vi "DS345_BurstMode.ProcCases.vi"(0 "i ref in":refnum<vi>, 1 "selector":string, 2 "Data":T1, 3 "call cluster":T2={"Object"="", "Selector"="", "CallType"=enum."synchronous", "Async Object"="", "Async Selector"="", "Data Descriptor"="", "Data"=[], "Error #"=0, "Expire"=0}, 5 "error in (no error)":errorcluster) -> (14 "i ref out":refnum<vi>, 17 "answer cluster":T2={"Object"="", "Selector"="", "CallType"=enum."synchronous", "Async Object"="", "Async Selector"="", "Data Descriptor"="", "Data"=[], "Error #"=0, "Expire"=0}, 19 "error out":errorcluster)   [LabVIEW 2014, in "DS345_BurstMode.lvlib"]
doc: "This method is called by a process from within the default case in the event loop. The methods of a class that are linked to events will be called from THIS method. Add your code here."
uses:
  DS345_BurstMode.lvlib
  CS_Core/CSSystem/CoreDefs/CoreDefs.call_type.ctl
  CS_Core/BaseProcess/BaseProcess.descriptor string definition.ctl
  CS_Core/CSSystem/CoreDefs/CoreDefs.rawDataType.ctl
  CS_Core/CSSystem/CoreLib/CoreLib.string 2 byte array.vi
  CS_Core/CSSystem/CoreLib/CoreLib.byte array 2 double.vi
  CS_Core/CSSystem/CoreLib/CoreLib.double 2 byte array.vi
  CS_Core/CSSystem/CoreLib/CoreLib.lvlib
  CS_Core/BaseProcess/BaseProcess.lvlib
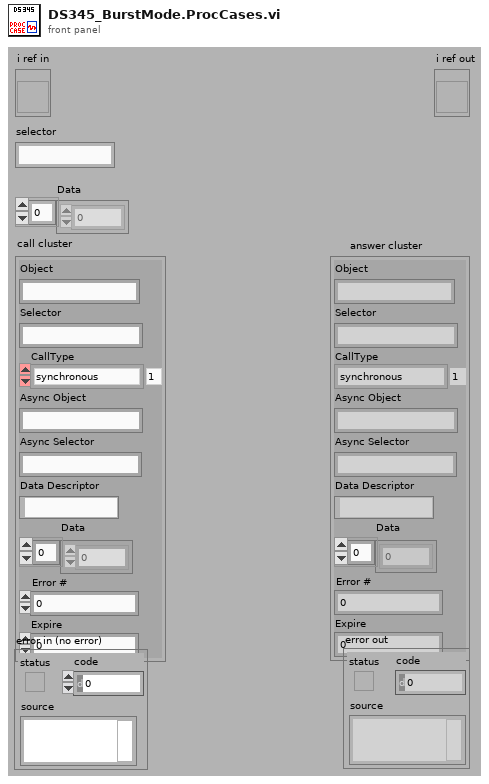
[diagram p1: front panel]
types:
  T1 = typedef "CoreDefs.rawDataType.ctl" = i8[]
  T2 = typedef "CoreDefs.call_type.ctl" = cluster{"Object":string, "Selector":string, "CallType":enum16{"simple", "synchronous", "asynchronous"}, "Async Object":string, "Async Selector":string, "Data Descriptor":T3, "Data":T1, "Error #":i32, "Expire":u32}
  T3 = typedef "BaseProcess.lvlib/BaseProcess.descriptor string definition.ctl" = string
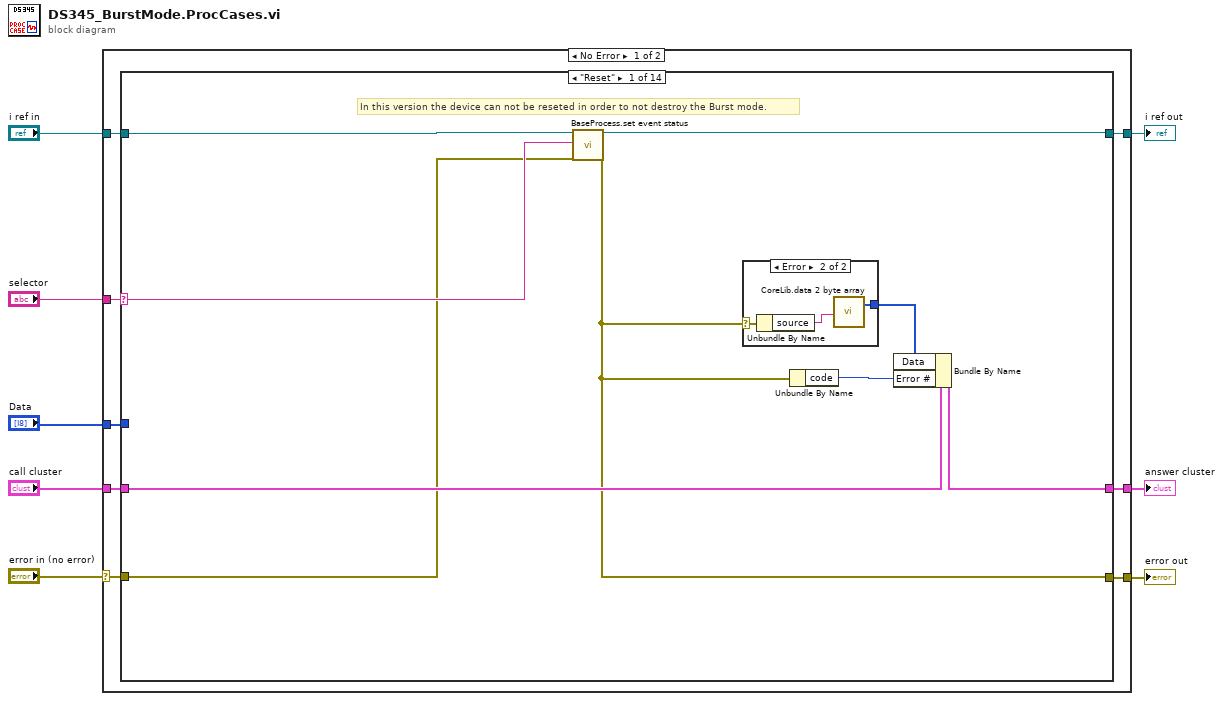
[diagram p0: block diagram]
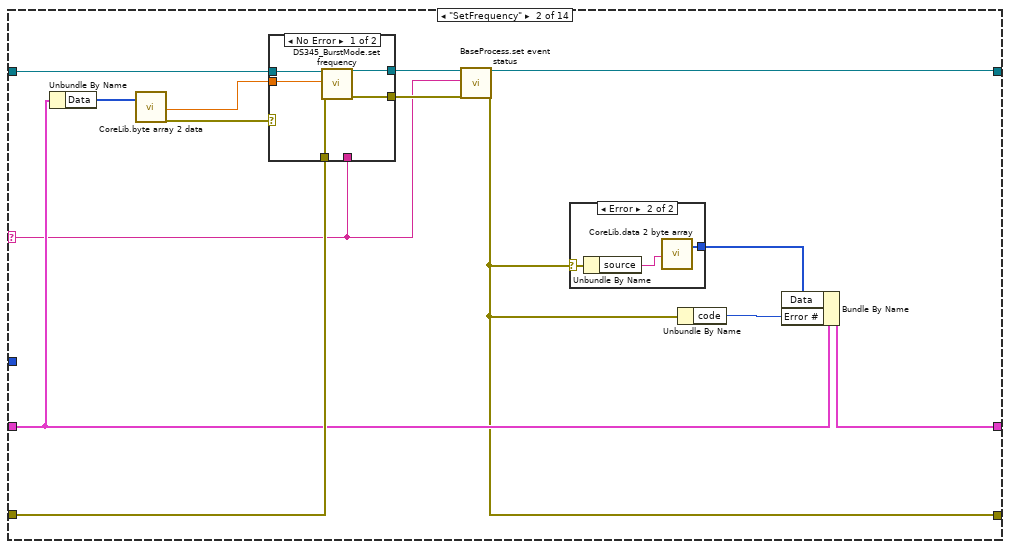
[diagram p3: hidden frame]
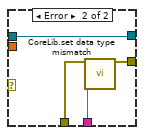
[diagram p5: hidden frame]
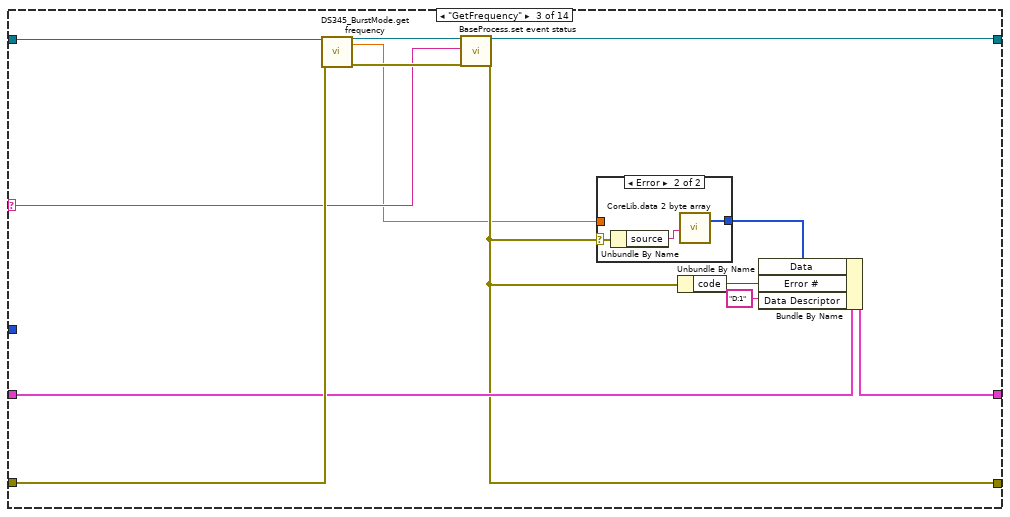
[diagram p6: hidden frame]
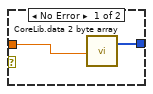
[diagram p7: hidden frame]
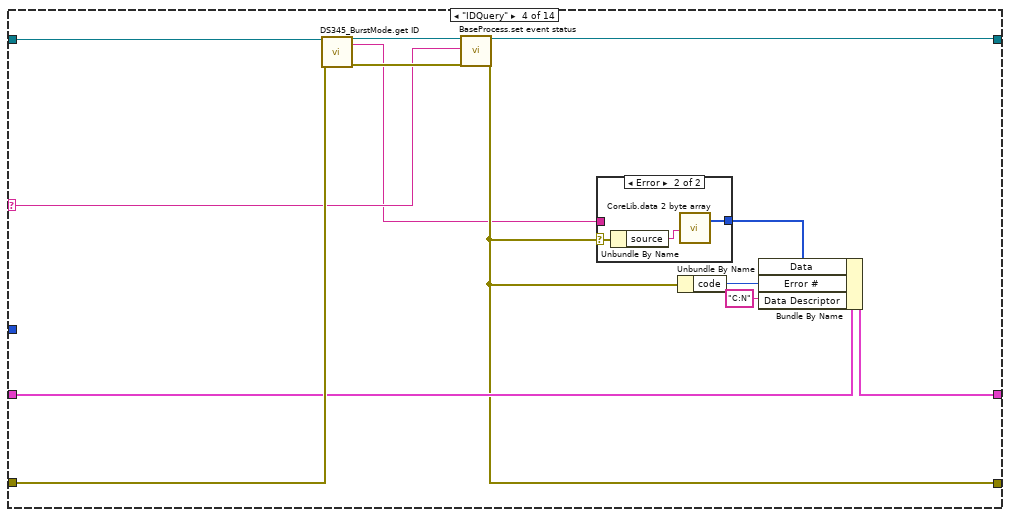
[diagram p8: hidden frame]
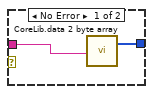
[diagram p9: hidden frame]
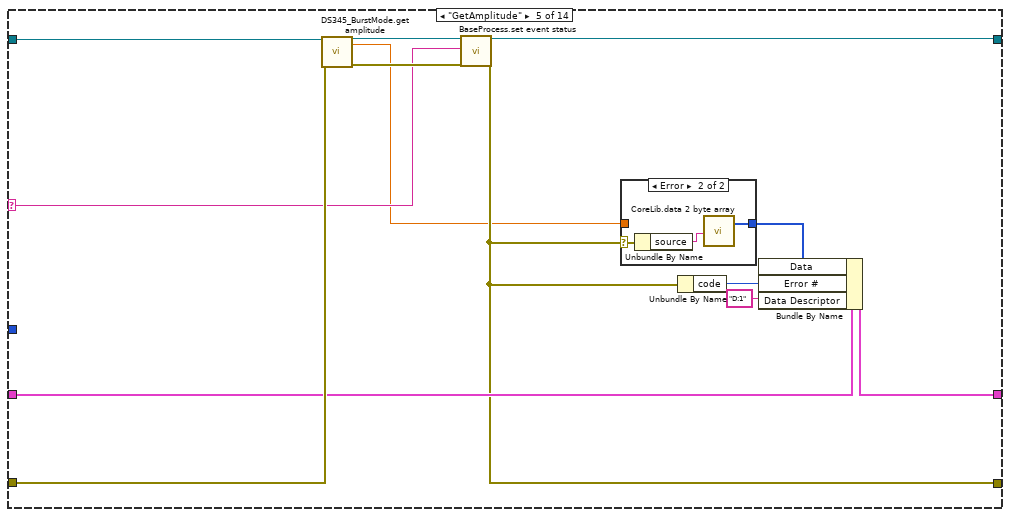
[diagram p10: hidden frame]
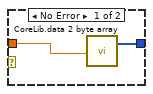
[diagram p11: hidden frame]
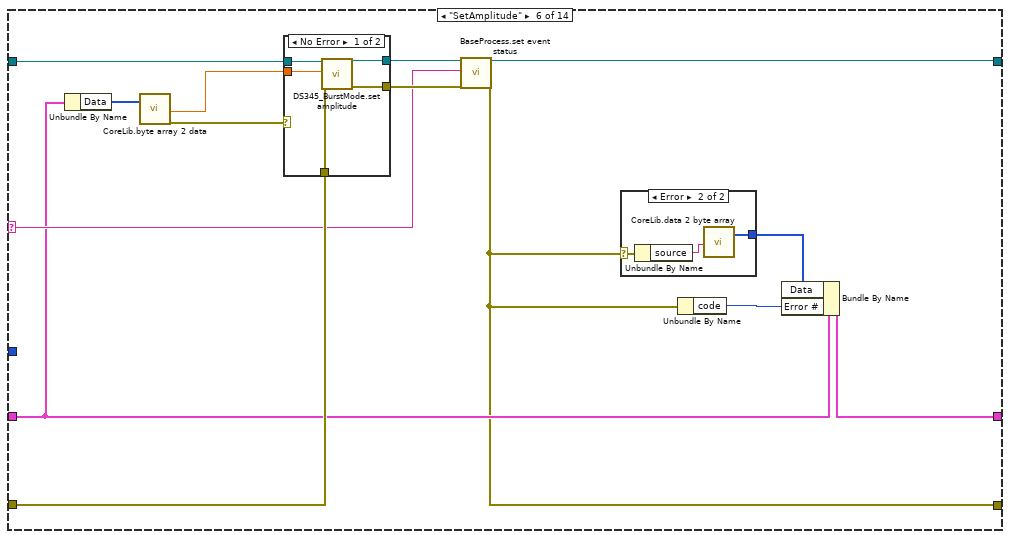
[diagram p12: hidden frame]
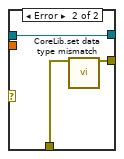
[diagram p14: hidden frame]
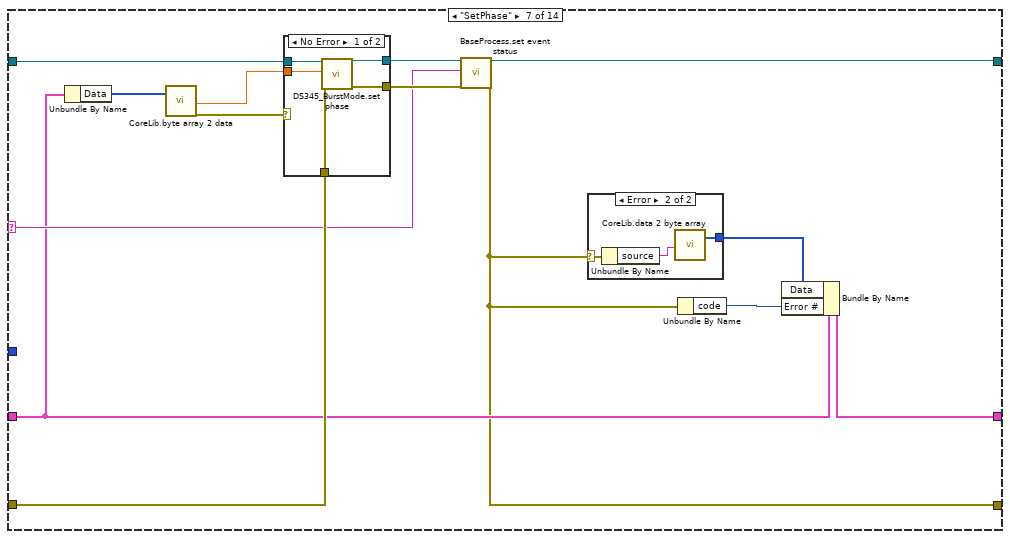
[diagram p15: hidden frame]
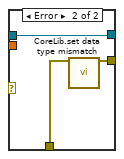
[diagram p17: hidden frame]
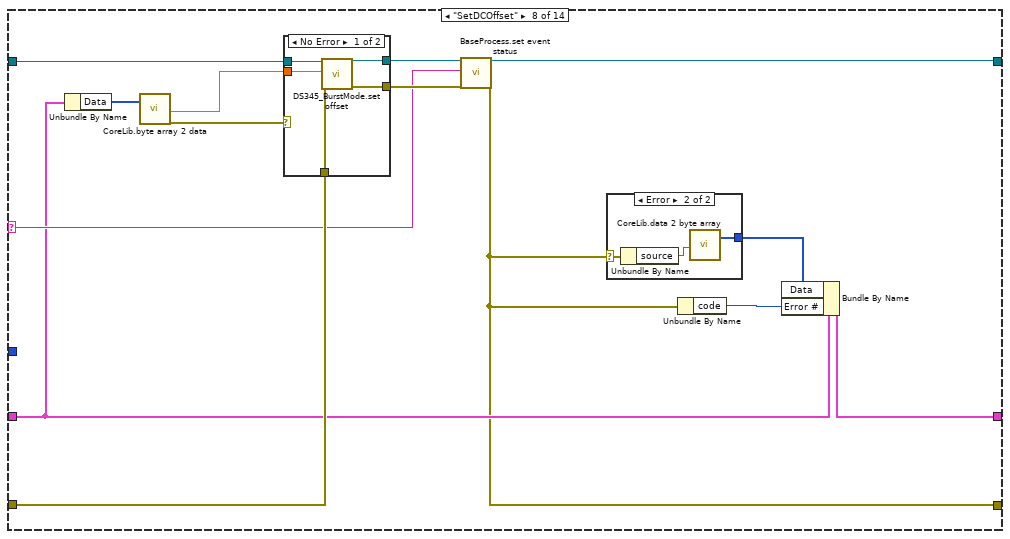
[diagram p18: hidden frame]
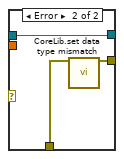
[diagram p20: hidden frame]
diagram:
  n1 = case shown="No Error" "error in (no error)" {
    selector: "error in (no error)" -> [w9 w345]
    tunnel: "selector" -> [w16 _]
    tunnel: [w15 w346] -> w7
    tunnel: "Data" -> [w14 _]
    tunnel: "call cluster" -> [w13 w346]
    tunnel: "i ref in" -> [w12 w347]
    tunnel: [w11 w347] -> w3
    tunnel: [w10 w345] -> w2
    frame No Error {
      n2 = case shown="\"Reset\"" w16 {
        selector: w16 -> [w21 w34 w59 w77 w95 w115 w140 w165 w190 w215 w240 w271 w313 w343]
        tunnel: w14 -> [_ _ _ _ _ _ _ _ _ _ _ _ _ w342]
        tunnel: w12 -> [w18 w40 w65 w83 w101 w120 w145 w170 w195 w220 w245 w276 w318 w337]
        tunnel: [w22 w37 w62 w80 w98 w117 w142 w167 w192 w217 w242 w273 w315 w344] -> w11
        tunnel: w13 -> [w25 w35 w60 w78 w96 w114 w139 w164 w189 w214 w239 w270 w312 w341]
        tunnel: [w24 w42 w67 w85 w103 w122 w147 w172 w197 w222 w247 w278 w320 w338] -> w15
        tunnel: w9 -> [w17 w39 w64 w82 w100 w119 w144 w169 w194 w219 w244 w275 w317 w340]
        tunnel: [w19 w33 w58 w76 w94 w113 w135 w160 w185 w210 w235 w260 w293 w339] -> w10
        frame "Reset" {
          # "In this version the device can not be reseted in order to not destroy the Burst mode."
          n3 = call "BaseProcess.set event status.vi"("i ref in"=w18, "EventStatus"=w21, "error in (no error)"=w17) -> ("i ref out"=w22:refnum<vi>, "error out"=w19:errorcluster)  [unwired: 14 in, 1 out]
          n4 = case shown="Error" w19 {
            selector: w19 -> [_ w28]
            tunnel: [_ w26] -> w20
            frame No Error {
            }
            frame Error {
              n5 = Unbundle By Name(w28) -> ("source"=w27:string)
              n6 = call-poly "CoreLib.data 2 byte array.vi"("string"=w27) -> ("byteArray out"=w26:T1)  [unwired: 18 in]
            }
          }
          n7 = Unbundle By Name(w19) -> ("code"=w23:i32)
          n8 = Bundle By Name(cluster=w25, "Data"=w20, "Error #"=w23) -> (w24:T2)
        }
        frame "SetFrequency" {
          n9 = Unbundle By Name(w35) -> ("Data"=w31:T1)
          n10 = call-poly "CoreLib.byte array 2 data.vi"("byteArray"=w31) -> ("d64"=w29:dbl, "error out"=w30:errorcluster)  [unwired: 16 in, 1 out]
          n11 = case shown="No Error" w30 {
            tunnel: w40 -> [w50 w54]
            tunnel: w39 -> [w49 w52]
            tunnel: [w48 w54] -> w38
            tunnel: [w47 w53] -> w36
            tunnel: w29 -> [w46 _]
            tunnel: w34 -> [_ w51]
            frame No Error {
              n12 = call "DS345_BurstMode.set frequency.vi"("i ref in"=w50, "frequency [Hz]"=w46, "error in (no error)"=w49) -> ("i ref out"=w48:refnum<vi>, "error out"=w47:errorcluster)  [unwired: 15 in]
            }
            frame Error {
              n13 = call "CoreLib.set data type mismatch.vi"("error in (no error)"=w52, "error source"=w51) -> ("error out"=w53:errorcluster)  [unwired: 17 in]
            }
          }
          n14 = call "BaseProcess.set event status.vi"("i ref in"=w38, "EventStatus"=w34, "error in (no error)"=w36) -> ("i ref out"=w37:refnum<vi>, "error out"=w33:errorcluster)  [unwired: 14 in, 1 out]
          n15 = case shown="Error" w33 {
            selector: w33 -> [_ w45]
            tunnel: [_ w43] -> w32
            frame No Error {
            }
            frame Error {
              n16 = Unbundle By Name(w45) -> ("source"=w44:string)
              n17 = call-poly "CoreLib.data 2 byte array.vi"("string"=w44) -> ("byteArray out"=w43:T1)  [unwired: 18 in]
            }
          }
          n18 = Unbundle By Name(w33) -> ("code"=w41:i32)
          n19 = Bundle By Name(cluster=w35, "Data"=w32, "Error #"=w41) -> (w42:T2)
        }
        frame "GetFrequency" {
          n20 = call "DS345_BurstMode.get frequency.vi"("i ref in"=w65, "error in (no error)"=w64) -> ("i ref out"=w63:refnum<vi>, "frequency [Hz}"=w56:dbl, "error out"=w61:errorcluster)  [unwired: 15 in]
          n21 = call "BaseProcess.set event status.vi"("i ref in"=w63, "EventStatus"=w59, "error in (no error)"=w61) -> ("i ref out"=w62:refnum<vi>, "error out"=w58:errorcluster)  [unwired: 14 in, 1 out]
          n22 = case shown="Error" w58 {
            selector: w58 -> [_ w72]
            tunnel: [w69 w70] -> w57
            tunnel: w56 -> [w68 _]
            frame No Error {
              n23 = call-poly "CoreLib.data 2 byte array.vi"("f64"=w68) -> ("byteArray out"=w69:T1)  [unwired: 18 in]
            }
            frame Error {
              n24 = Unbundle By Name(w72) -> ("source"=w71:string)
              n25 = call-poly "CoreLib.data 2 byte array.vi"("string"=w71) -> ("byteArray out"=w70:T1)  [unwired: 18 in]
            }
          }
          n26 = Unbundle By Name(w58) -> ("code"=w66:i32)
          n27 = Bundle By Name(cluster=w60, "Data"=w57, "Error #"=w66, "Data Descriptor"="D:1") -> (w67:T2)
        }
        frame "IDQuery" {
          n28 = call "DS345_BurstMode.get ID.vi"("i ref in"=w83, "error in (no error)"=w82) -> ("i ref out"=w81:refnum<vi>, "instrumentID"=w74:string, "error out"=w79:errorcluster)  [unwired: 15 in]
          n29 = call "BaseProcess.set event status.vi"("i ref in"=w81, "EventStatus"=w77, "error in (no error)"=w79) -> ("i ref out"=w80:refnum<vi>, "error out"=w76:errorcluster)  [unwired: 14 in, 1 out]
          n30 = case shown="Error" w76 {
            selector: w76 -> [_ w90]
            tunnel: [w87 w88] -> w75
            tunnel: w74 -> [w86 _]
            frame No Error {
              n31 = call-poly "CoreLib.data 2 byte array.vi"("string"=w86) -> ("byteArray out"=w87:T1)  [unwired: 18 in]
            }
            frame Error {
              n32 = Unbundle By Name(w90) -> ("source"=w89:string)
              n33 = call-poly "CoreLib.data 2 byte array.vi"("string"=w89) -> ("byteArray out"=w88:T1)  [unwired: 18 in]
            }
          }
          n34 = Unbundle By Name(w76) -> ("code"=w84:i32)
          n35 = Bundle By Name(cluster=w78, "Data"=w75, "Error #"=w84, "Data Descriptor"="C:N") -> (w85:T2)
        }
        frame "GetAmplitude" {
          n36 = call "DS345_BurstMode.get amplitude.vi"("i ref in"=w101, "error in (no error)"=w100) -> ("i ref out"=w99:refnum<vi>, "amplitude [V]"=w91:dbl, "error out"=w97:errorcluster)  [unwired: 15 in]
          n37 = call "BaseProcess.set event status.vi"("i ref in"=w99, "EventStatus"=w95, "error in (no error)"=w97) -> ("i ref out"=w98:refnum<vi>, "error out"=w94:errorcluster)  [unwired: 14 in, 1 out]
          n38 = case shown="Error" w94 {
            selector: w94 -> [_ w108]
            tunnel: [w105 w106] -> w93
            tunnel: w91 -> [w104 _]
            frame No Error {
              n39 = call-poly "CoreLib.data 2 byte array.vi"("f64"=w104) -> ("byteArray out"=w105:T1)  [unwired: 18 in]
            }
            frame Error {
              n40 = Unbundle By Name(w108) -> ("source"=w107:string)
              n41 = call-poly "CoreLib.data 2 byte array.vi"("string"=w107) -> ("byteArray out"=w106:T1)  [unwired: 18 in]
            }
          }
          n42 = Unbundle By Name(w94) -> ("code"=w102:i32)
          n43 = Bundle By Name(cluster=w96, "Data"=w93, "Error #"=w102, "Data Descriptor"="D:1") -> (w103:T2)
        }
        frame "SetAmplitude" {
          n44 = Unbundle By Name(w114) -> ("Data"=w111:T1)
          n45 = call-poly "CoreLib.byte array 2 data.vi"("byteArray"=w111) -> ("d64"=w109:dbl, "error out"=w110:errorcluster)  [unwired: 16 in, 1 out]
          n46 = case shown="No Error" w110 {
            tunnel: w120 -> [w130 w133]
            tunnel: w119 -> [w129 w131]
            tunnel: [w128 w133] -> w118
            tunnel: [w127 w132] -> w116
            tunnel: w109 -> [w126 _]
            frame No Error {
              n47 = call "DS345_BurstMode.set amplitude.vi"("i ref in"=w130, "amplitude [V]"=w126, "error in (no error)"=w129) -> ("i ref out"=w128:refnum<vi>, "error out"=w127:errorcluster)  [unwired: 15 in]
            }
            frame Error {
              n48 = call "CoreLib.set data type mismatch.vi"("error in (no error)"=w131) -> ("error out"=w132:errorcluster)  [unwired: 18 in]
            }
          }
          n49 = call "BaseProcess.set event status.vi"("i ref in"=w118, "EventStatus"=w115, "error in (no error)"=w116) -> ("i ref out"=w117:refnum<vi>, "error out"=w113:errorcluster)  [unwired: 14 in, 1 out]
          n50 = case shown="Error" w113 {
            selector: w113 -> [_ w125]
            tunnel: [_ w123] -> w112
            frame No Error {
            }
            frame Error {
              n51 = Unbundle By Name(w125) -> ("source"=w124:string)
              n52 = call-poly "CoreLib.data 2 byte array.vi"("string"=w124) -> ("byteArray out"=w123:T1)  [unwired: 18 in]
            }
          }
          n53 = Unbundle By Name(w113) -> ("code"=w121:i32)
          n54 = Bundle By Name(cluster=w114, "Data"=w112, "Error #"=w121) -> (w122:T2)
        }
        frame "SetPhase" {
          n55 = Unbundle By Name(w139) -> ("Data"=w138:T1)
          n56 = call-poly "CoreLib.byte array 2 data.vi"("byteArray"=w138) -> ("d64"=w136:dbl, "error out"=w137:errorcluster)  [unwired: 16 in, 1 out]
          n57 = case shown="No Error" w137 {
            tunnel: w145 -> [w155 w158]
            tunnel: w144 -> [w154 w156]
            tunnel: [w153 w158] -> w143
            tunnel: [w152 w157] -> w141
            tunnel: w136 -> [w151 _]
            frame No Error {
              n58 = call "DS345_BurstMode.set phase.vi"("i ref in"=w155, "phase [degree]"=w151, "error in (no error)"=w154) -> ("i ref out"=w153:refnum<vi>, "error out"=w152:errorcluster)  [unwired: 15 in]
            }
            frame Error {
              n59 = call "CoreLib.set data type mismatch.vi"("error in (no error)"=w156) -> ("error out"=w157:errorcluster)  [unwired: 18 in]
            }
          }
          n60 = call "BaseProcess.set event status.vi"("i ref in"=w143, "EventStatus"=w140, "error in (no error)"=w141) -> ("i ref out"=w142:refnum<vi>, "error out"=w135:errorcluster)  [unwired: 14 in, 1 out]
          n61 = case shown="Error" w135 {
            selector: w135 -> [_ w150]
            tunnel: [_ w148] -> w134
            frame No Error {
            }
            frame Error {
              n62 = Unbundle By Name(w150) -> ("source"=w149:string)
              n63 = call-poly "CoreLib.data 2 byte array.vi"("string"=w149) -> ("byteArray out"=w148:T1)  [unwired: 18 in]
            }
          }
          n64 = Unbundle By Name(w135) -> ("code"=w146:i32)
          n65 = Bundle By Name(cluster=w139, "Data"=w134, "Error #"=w146) -> (w147:T2)
        }
        frame "SetDCOffset" {
          n66 = Unbundle By Name(w164) -> ("Data"=w163:T1)
          n67 = call-poly "CoreLib.byte array 2 data.vi"("byteArray"=w163) -> ("d64"=w161:dbl, "error out"=w162:errorcluster)  [unwired: 16 in, 1 out]
          n68 = case shown="No Error" w162 {
            tunnel: w170 -> [w180 w183]
            tunnel: w169 -> [w179 w181]
            tunnel: [w178 w183] -> w168
            tunnel: [w177 w182] -> w166
            tunnel: w161 -> [w176 _]
            frame No Error {
              n69 = call "DS345_BurstMode.set offset.vi"("i ref in"=w180, "offset [V]"=w176, "error in (no error)"=w179) -> ("i ref out"=w178:refnum<vi>, "error out"=w177:errorcluster)  [unwired: 15 in]
            }
            frame Error {
              n70 = call "CoreLib.set data type mismatch.vi"("error in (no error)"=w181) -> ("error out"=w182:errorcluster)  [unwired: 18 in]
            }
          }
          n71 = call "BaseProcess.set event status.vi"("i ref in"=w168, "EventStatus"=w165, "error in (no error)"=w166) -> ("i ref out"=w167:refnum<vi>, "error out"=w160:errorcluster)  [unwired: 14 in, 1 out]
          n72 = case shown="Error" w160 {
            selector: w160 -> [_ w175]
            tunnel: [_ w173] -> w159
            frame No Error {
            }
            frame Error {
              n73 = Unbundle By Name(w175) -> ("source"=w174:string)
              n74 = call-poly "CoreLib.data 2 byte array.vi"("string"=w174) -> ("byteArray out"=w173:T1)  [unwired: 18 in]
            }
          }
          n75 = Unbundle By Name(w160) -> ("code"=w171:i32)
          n76 = Bundle By Name(cluster=w164, "Data"=w159, "Error #"=w171) -> (w172:T2)
        }
        frame "SetDelay" {
          n77 = Unbundle By Name(w189) -> ("Data"=w188:T1)
          n78 = call-poly "CoreLib.byte array 2 data.vi"("byteArray"=w188) -> ("d64"=w186:dbl, "error out"=w187:errorcluster)  [unwired: 16 in, 1 out]
          n79 = case shown="No Error" w187 {
            tunnel: w195 -> [w205 w208]
            tunnel: w194 -> [w204 w206]
            tunnel: [w203 w208] -> w193
            tunnel: [w202 w207] -> w191
            tunnel: w186 -> [w201 _]
            frame No Error {
              n80 = call "DS345_BurstMode.set delay.vi"("i ref in"=w205, "delay [us]"=w201, "error in (no error)"=w204) -> ("i ref out"=w203:refnum<vi>, "error out"=w202:errorcluster)  [unwired: 15 in]
            }
            frame Error {
              n81 = call "CoreLib.set data type mismatch.vi"("error in (no error)"=w206) -> ("error out"=w207:errorcluster)  [unwired: 18 in]
            }
          }
          n82 = call "BaseProcess.set event status.vi"("i ref in"=w193, "EventStatus"=w190, "error in (no error)"=w191) -> ("i ref out"=w192:refnum<vi>, "error out"=w185:errorcluster)  [unwired: 14 in, 1 out]
          n83 = case shown="Error" w185 {
            selector: w185 -> [_ w200]
            tunnel: [_ w198] -> w184
            frame No Error {
            }
            frame Error {
              n84 = Unbundle By Name(w200) -> ("source"=w199:string)
              n85 = call-poly "CoreLib.data 2 byte array.vi"("string"=w199) -> ("byteArray out"=w198:T1)  [unwired: 18 in]
            }
          }
          n86 = Unbundle By Name(w185) -> ("code"=w196:i32)
          n87 = Bundle By Name(cluster=w189, "Data"=w184, "Error #"=w196) -> (w197:T2)
        }
        frame "SetGate" {
          n88 = Unbundle By Name(w214) -> ("Data"=w213:T1)
          n89 = call-poly "CoreLib.byte array 2 data.vi"("byteArray"=w213) -> ("d64"=w212:dbl, "error out"=w211:errorcluster)  [unwired: 16 in, 1 out]
          n90 = case shown="No Error" w211 {
            tunnel: w220 -> [w230 w233]
            tunnel: w219 -> [w229 w231]
            tunnel: [w228 w233] -> w218
            tunnel: [w227 w232] -> w216
            tunnel: w212 -> [w226 _]
            frame No Error {
              n91 = call "DS345_BurstMode.set gate.vi"("i ref in"=w230, "gate [us]"=w226, "error in (no error)"=w229) -> ("i ref out"=w228:refnum<vi>, "error out"=w227:errorcluster)  [unwired: 15 in]
            }
            frame Error {
              n92 = call "CoreLib.set data type mismatch.vi"("error in (no error)"=w231) -> ("error out"=w232:errorcluster)  [unwired: 18 in]
            }
          }
          n93 = call "BaseProcess.set event status.vi"("i ref in"=w218, "EventStatus"=w215, "error in (no error)"=w216) -> ("i ref out"=w217:refnum<vi>, "error out"=w210:errorcluster)  [unwired: 14 in, 1 out]
          n94 = case shown="Error" w210 {
            selector: w210 -> [_ w225]
            tunnel: [_ w223] -> w209
            frame No Error {
            }
            frame Error {
              n95 = Unbundle By Name(w225) -> ("source"=w224:string)
              n96 = call-poly "CoreLib.data 2 byte array.vi"("string"=w224) -> ("byteArray out"=w223:T1)  [unwired: 18 in]
            }
          }
          n97 = Unbundle By Name(w210) -> ("code"=w221:i32)
          n98 = Bundle By Name(cluster=w214, "Data"=w209, "Error #"=w221) -> (w222:T2)
        }
        frame "SetGauss" {
          n99 = Unbundle By Name(w239) -> ("Data"=w238:T1)
          n100 = call-poly "CoreLib.byte array 2 data.vi"("byteArray"=w238) -> ("d64"=w236:dbl, "error out"=w237:errorcluster)  [unwired: 16 in, 1 out]
          n101 = case shown="No Error" w237 {
            tunnel: w245 -> [w255 w258]
            tunnel: w244 -> [w254 w256]
            tunnel: [w253 w258] -> w243
            tunnel: [w252 w257] -> w241
            tunnel: w236 -> [w251 _]
            frame No Error {
              n102 = call "DS345_BurstMode.set gauss.vi"("i ref in"=w255, "length [us]"=w251, "error in (no error)"=w254) -> ("i ref out"=w253:refnum<vi>, "error out"=w252:errorcluster)  [unwired: 15 in]
            }
            frame Error {
              n103 = call "CoreLib.set data type mismatch.vi"("error in (no error)"=w256) -> ("error out"=w257:errorcluster)  [unwired: 18 in]
            }
          }
          n104 = call "BaseProcess.set event status.vi"("i ref in"=w243, "EventStatus"=w240, "error in (no error)"=w241) -> ("i ref out"=w242:refnum<vi>, "error out"=w235:errorcluster)  [unwired: 14 in, 1 out]
          n105 = case shown="Error" w235 {
            selector: w235 -> [_ w250]
            tunnel: [_ w248] -> w234
            frame No Error {
            }
            frame Error {
              n106 = Unbundle By Name(w250) -> ("source"=w249:string)
              n107 = call-poly "CoreLib.data 2 byte array.vi"("string"=w249) -> ("byteArray out"=w248:T1)  [unwired: 18 in]
            }
          }
          n108 = Unbundle By Name(w235) -> ("code"=w246:i32)
          n109 = Bundle By Name(cluster=w239, "Data"=w234, "Error #"=w246) -> (w247:T2)
        }
        frame "SetDelayGate" {
          n110 = Unbundle By Name(w270) -> ("Data"=w269:T1)
          n111 = call-poly "CoreLib.byte array 2 data.vi"("byteArray"=w269) -> ("byteArray out"=w268:T1, "d64"=w263:dbl, "error out"=w266:errorcluster)  [unwired: 16 in]
          n112 = call-poly "CoreLib.byte array 2 data.vi"("byteArray"=w268, "error in (no error)"=w266) -> ("byteArray out"=w267:T1, "d64"=w262:dbl, "error out"=w265:errorcluster)  [unwired: 15 in]
          n113 = call-poly "CoreLib.byte array 2 data.vi"("byteArray"=w267, "error in (no error)"=w265) -> ("d64"=w261:dbl, "error out"=w264:errorcluster)  [unwired: 15 in, 1 out]
          n114 = case shown="Error" w264 {
            tunnel: w276 -> [w288 w291]
            tunnel: w275 -> [w285 w289]
            tunnel: [w287 w291] -> w274
            tunnel: [w286 w290] -> w272
            tunnel: w263 -> [w284 _]
            tunnel: w262 -> [w283 _]
            tunnel: w261 -> [w282 _]
            frame No Error {
              n115 = call "DS345_BurstMode.set delay gate.vi"("i ref in"=w288, "sampleFrequency [Hz]"=w284, "delay [us]"=w283, "gate [us]"=w282, "error in (no error)"=w285) -> ("i ref out"=w287:refnum<vi>, "error out"=w286:errorcluster)  [unwired: 13 in]
            }
            frame Error {
              n116 = call "CoreLib.set data type mismatch.vi"("error in (no error)"=w289) -> ("error out"=w290:errorcluster)  [unwired: 18 in]
            }
          }
          n117 = call "BaseProcess.set event status.vi"("i ref in"=w274, "EventStatus"=w271, "error in (no error)"=w272) -> ("i ref out"=w273:refnum<vi>, "error out"=w260:errorcluster)  [unwired: 14 in, 1 out]
          n118 = case shown="Error" w260 {
            selector: w260 -> [_ w281]
            tunnel: [_ w279] -> w259
            frame No Error {
            }
            frame Error {
              n119 = Unbundle By Name(w281) -> ("source"=w280:string)
              n120 = call-poly "CoreLib.data 2 byte array.vi"("string"=w280) -> ("byteArray out"=w279:T1)  [unwired: 18 in]
            }
          }
          n121 = Unbundle By Name(w260) -> ("code"=w277:i32)
          n122 = Bundle By Name(cluster=w270, "Data"=w259, "Error #"=w277) -> (w278:T2)
        }
        frame "SetRamp" {
          n123 = Unbundle By Name(w312) -> ("Data"=w311:T1)
          n124 = call-poly "CoreLib.byte array 2 data.vi"("byteArray"=w311) -> ("byteArray out"=w310:T1, "d64"=w299:dbl, "error out"=w305:errorcluster)  [unwired: 16 in]
          n125 = call-poly "CoreLib.byte array 2 data.vi"("byteArray"=w310, "error in (no error)"=w305) -> ("byteArray out"=w309:T1, "d64"=w298:dbl, "error out"=w304:errorcluster)  [unwired: 15 in]
          n126 = call-poly "CoreLib.byte array 2 data.vi"("byteArray"=w309, "error in (no error)"=w304) -> ("byteArray out"=w308:T1, "d64"=w297:dbl, "error out"=w303:errorcluster)  [unwired: 15 in]
          n127 = call-poly "CoreLib.byte array 2 data.vi"("byteArray"=w308, "error in (no error)"=w303) -> ("byteArray out"=w307:T1, "d64"=w296:dbl, "error out"=w302:errorcluster)  [unwired: 15 in]
          n128 = call-poly "CoreLib.byte array 2 data.vi"("byteArray"=w307, "error in (no error)"=w302) -> ("byteArray out"=w306:T1, "d64"=w295:dbl, "error out"=w301:errorcluster)  [unwired: 15 in]
          n129 = call-poly "CoreLib.byte array 2 data.vi"("byteArray"=w306, "error in (no error)"=w301) -> ("d64"=w294:dbl, "error out"=w300:errorcluster)  [unwired: 15 in, 1 out]
          n130 = case shown="Error" w300 {
            tunnel: w318 -> [w333 w336]
            tunnel: w317 -> [w330 w334]
            tunnel: [w332 w336] -> w316
            tunnel: [w331 w335] -> w314
            tunnel: w299 -> [w329 _]
            tunnel: w298 -> [w328 _]
            tunnel: w297 -> [w326 _]
            tunnel: w296 -> [w327 _]
            tunnel: w295 -> [w325 _]
            tunnel: w294 -> [w324 _]
            frame No Error {
              n131 = call "DS345_BurstMode.set ramp.vi"("i ref in"=w333, "sampleFrequency [Hz]"=w329, "delay [us]"=w328, "error in (no error)"=w330, "x1 [us]"=w326, "x2 [us]"=w325, "y1 [V]"=w327, "y2 [V]"=w324) -> ("i ref out"=w332:refnum<vi>, "error out"=w331:errorcluster)  [unwired: 10 in]
            }
            frame Error {
              n132 = call "CoreLib.set data type mismatch.vi"("error in (no error)"=w334) -> ("error out"=w335:errorcluster)  [unwired: 18 in]
            }
          }
          n133 = call "BaseProcess.set event status.vi"("i ref in"=w316, "EventStatus"=w313, "error in (no error)"=w314) -> ("i ref out"=w315:refnum<vi>, "error out"=w293:errorcluster)  [unwired: 14 in, 1 out]
          n134 = case shown="Error" w293 {
            selector: w293 -> [_ w323]
            tunnel: [_ w321] -> w292
            frame No Error {
            }
            frame Error {
              n135 = Unbundle By Name(w323) -> ("source"=w322:string)
              n136 = call-poly "CoreLib.data 2 byte array.vi"("string"=w322) -> ("byteArray out"=w321:T1)  [unwired: 18 in]
            }
          }
          n137 = Unbundle By Name(w293) -> ("code"=w319:i32)
          n138 = Bundle By Name(cluster=w312, "Data"=w292, "Error #"=w319) -> (w320:T2)
        }
        frame Default {
          # "make sure attribute data\nare kept in memory"
          n139 = call "DS345_BurstMode.get i attribute.vi"("i ref in"=w337) -> ()  [unwired: 16 in, 3 out]
          n140 = call "BaseProcess.ProcCases.vi"("i ref in"=w337, "selector"=w343, "Data"=w342, "call cluster"=w341, "error in (no error)"=w340) -> ("i ref out"=w344:refnum<vi>, "answer cluster"=w338:T2, "error out"=w339:errorcluster)  [unwired: 12 in]
        }
      }
    }
    frame Error {
    }
  }
  "answer cluster" <- w7
  "i ref out" <- w3
  "error out" <- w2
